vi "Untitled 1.vi"() -> ()   [LabVIEW 2023]
uses:
  Control Timer.ctl
panel:
  out "State":string
  out "RELEASE ALL":bool
  out "MXING":bool
  out "BOILING MILK":bool
  out "ADDING MILK":bool
  out "BOILING":bool
  out "ADDING COFFEE":bool
  out "ADDING WATER":bool
  in  "STOP":bool
  in  "WHITE COFFEE":bool
  in  "CAPUCCINO":bool
  in  "ESPRESSO LONG":bool
  in  "ESPRESSO SHORT":bool
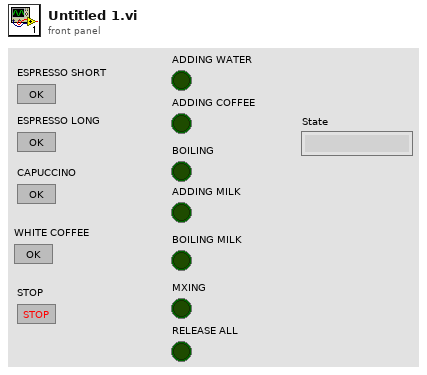
[diagram p1: front panel]
types:
  T1 = typedef "Control Timer.ctl" = enum16{"Timecheck", "Reset"}
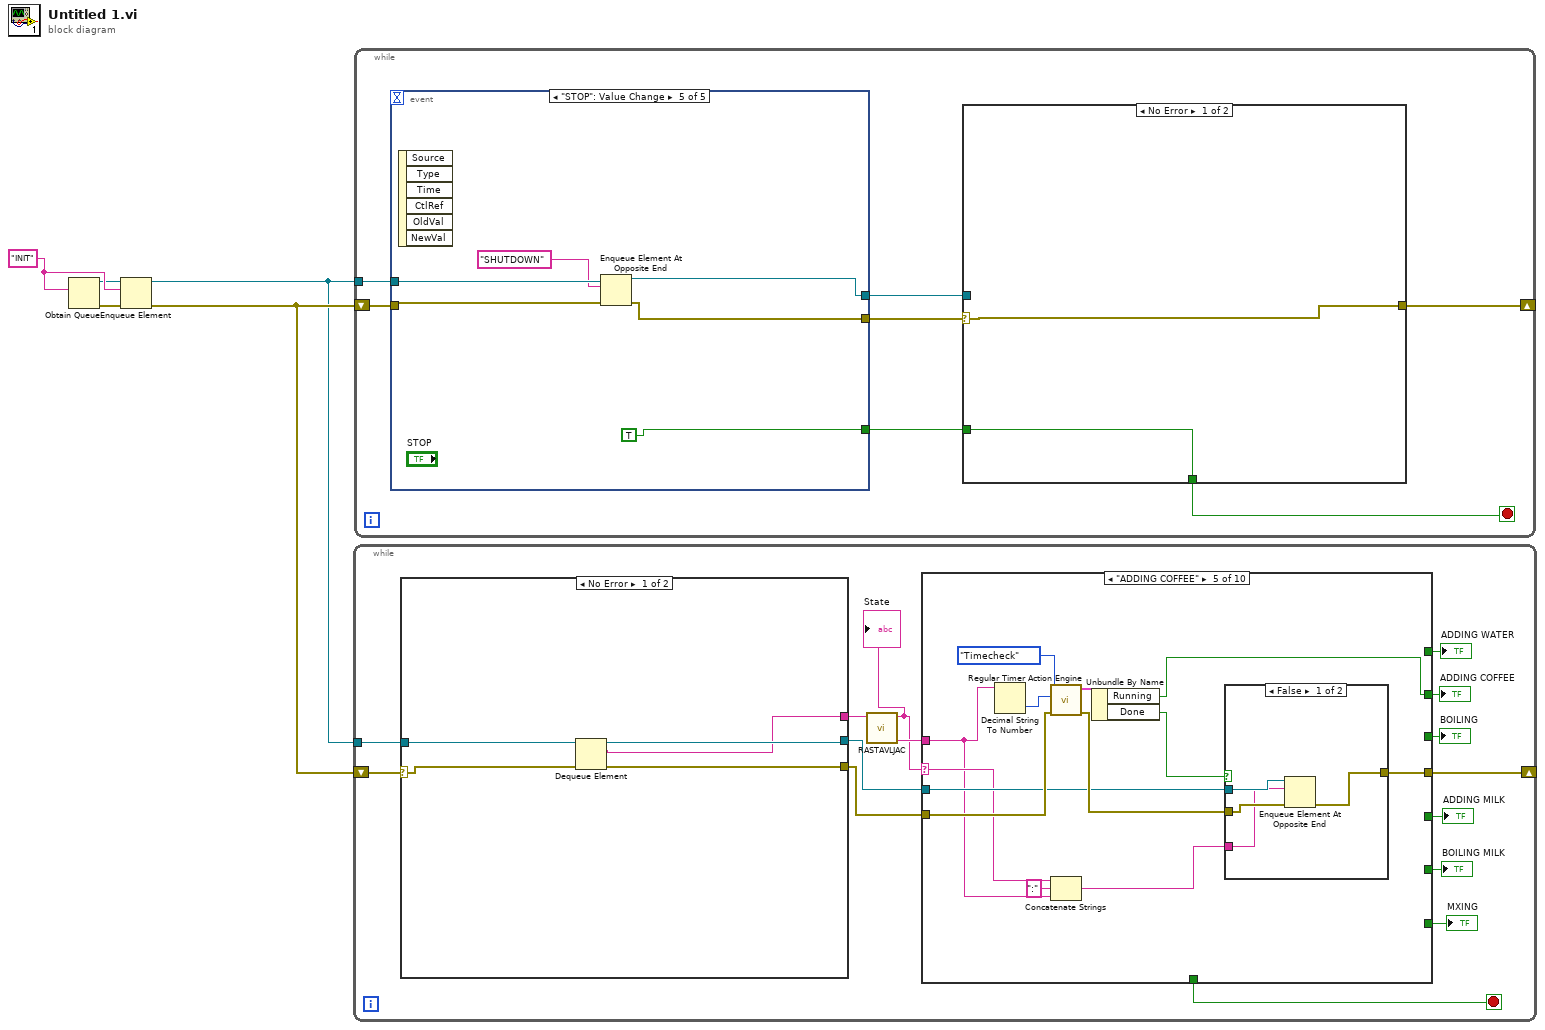
[diagram p0: block diagram]
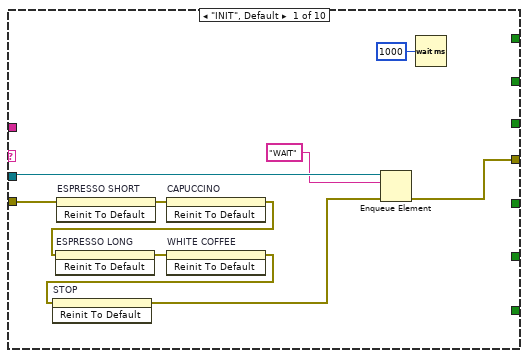
[diagram p2: hidden frame]
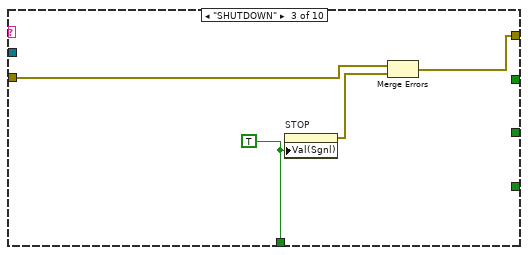
[diagram p4: hidden frame]
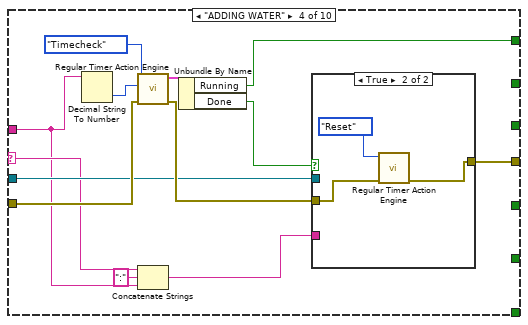
[diagram p5: hidden frame]
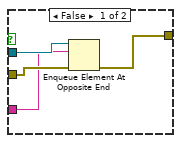
[diagram p6: hidden frame]
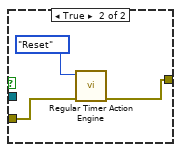
[diagram p7: hidden frame]
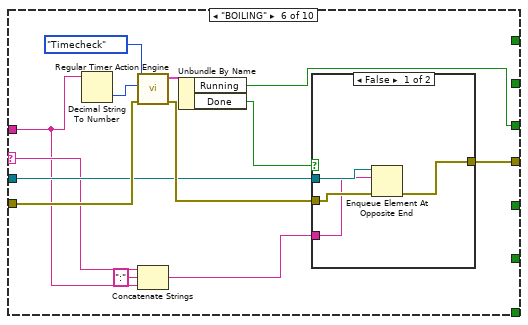
[diagram p8: hidden frame]
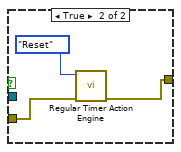
[diagram p9: hidden frame]
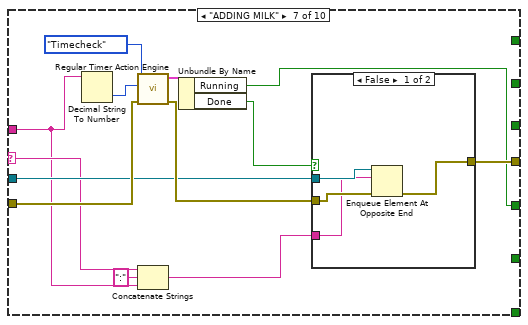
[diagram p10: hidden frame]
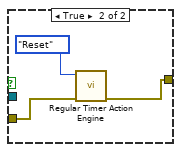
[diagram p11: hidden frame]
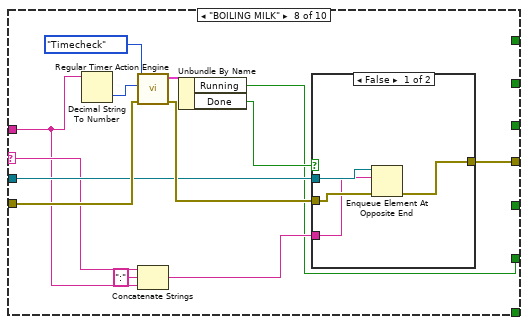
[diagram p12: hidden frame]
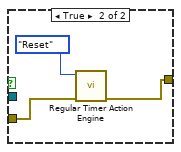
[diagram p13: hidden frame]
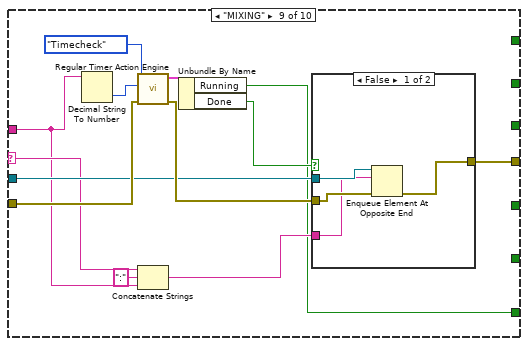
[diagram p14: hidden frame]
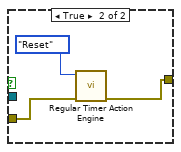
[diagram p15: hidden frame]
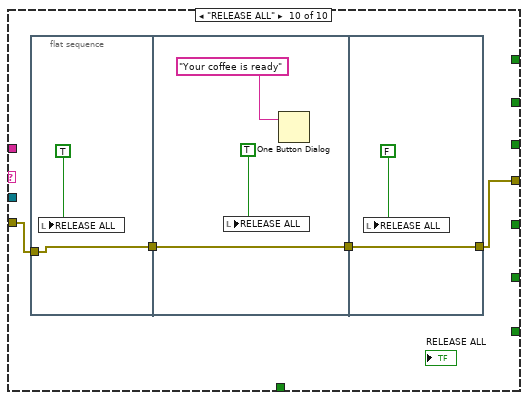
[diagram p16: hidden frame]
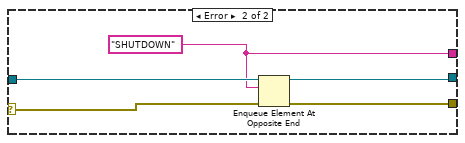
[diagram p17: hidden frame]
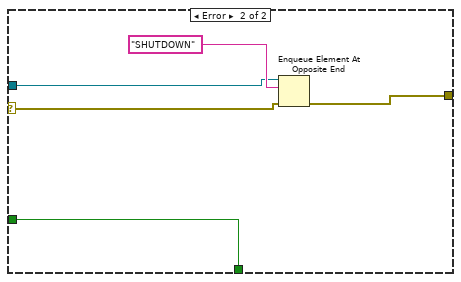
[diagram p18: hidden frame]
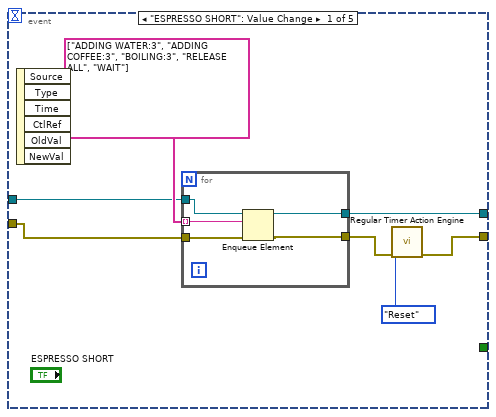
[diagram p19: hidden frame]
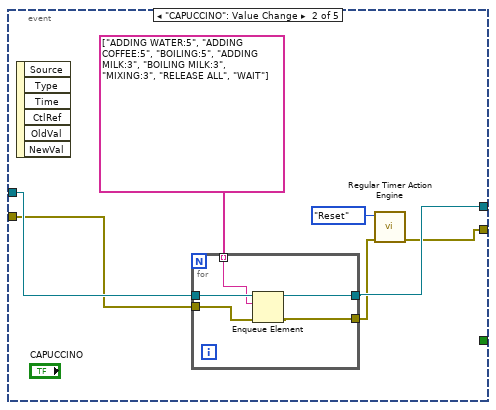
[diagram p20: hidden frame]
diagram:
  w4 = "INIT"
  n1 = Obtain Queue(element data type=w4) -> (queue out=w3:refnum<queue>, error out=w5:errorcluster)  [unwired: 4 in, 1 out]
  n2 = Enqueue Element(queue=w3, element=w4, error in (no error)=w5) -> (queue out=w1:refnum<queue>, error out=w2:errorcluster)  [unwired: 1 in, 1 out]
  n3 = while {
    tunnel: w1 -> [w19]
    shift-right: [w13] -> _
    shift-left: w2 -> [w20]
    stop <- w12 stop-if-true
    n4 = case shown="No Error" w20 {
      selector: w20 -> [w170 w176]
      tunnel: w19 -> [w171 w175]
      tunnel: [w169 w173] -> w15
      tunnel: [w168 w174] -> w14
      tunnel: [w167 w172] -> w18
      frame No Error {
        n5 = Dequeue Element(queue=w171, error in (no error)=w170) -> (queue out=w168:refnum<queue>, element=w167:string, error out=w169:errorcluster)  [unwired: 1 in, 1 out]
      }
      frame Error {
        w172 = "SHUTDOWN"
        n6 = Enqueue Element At Opposite End(queue=w175, element=w172, error in (no error)=w176) -> (queue out=w174:refnum<queue>, error out=w173:errorcluster)  [unwired: 1 in, 1 out]
      }
    }
    n7 = call "RASTAVLJAC.vi"("Input"=w18) -> ("Argument"=w17:string, "State"=w16:string)  [unwired: 9 in]
    "State" <- w16
    n8 = case shown="\"ADDING COFFEE\"" w16 {
      selector: w16 -> [_ _ _ w39 w60 w80 w100 w120 w140 _]
      tunnel: w17 -> [_ _ _ w38 w59 w79 w99 w119 w139 _]
      tunnel: w15 -> [w27 w31 w33 w46 w66 w86 w106 w126 w146 w159]
      tunnel: w14 -> [w30 _ _ w40 w61 w81 w101 w121 w141 _]
      tunnel: [w28 w31 w32 w41 w62 w82 w102 w122 w142 w156] -> w13
      tunnel: [_ _ w35 _ _ _ _ _ _ _] -> w12
      tunnel: [_ _ _ w44 _ _ _ _ _ _] -> w11
      tunnel: [_ _ _ _ w56 _ _ _ _ _] -> w10
      tunnel: [_ _ _ _ _ w76 _ _ _ _] -> w9
      tunnel: [_ _ _ _ _ _ w96 _ _ _] -> w8
      tunnel: [_ _ _ _ _ _ _ w116 _ _] -> w7
      tunnel: [_ _ _ _ _ _ _ _ w136 _] -> w6
      frame "INIT", Default {
        n9 = invoke on="ESPRESSO SHORT" class="Bool" method="Reinit To Default"(error in=w27) -> (error out=w26:errorcluster)  [unwired: 2 in, 2 out]
        n10 = invoke on="CAPUCCINO" class="Bool" method="Reinit To Default"(error in=w26) -> (error out=w25:errorcluster)  [unwired: 2 in, 2 out]
        n11 = invoke on="ESPRESSO LONG" class="Bool" method="Reinit To Default"(error in=w25) -> (error out=w24:errorcluster)  [unwired: 2 in, 2 out]
        n12 = invoke on="WHITE COFFEE" class="Bool" method="Reinit To Default"(error in=w24) -> (error out=w23:errorcluster)  [unwired: 2 in, 2 out]
        n13 = invoke on="STOP" class="Bool" method="Reinit To Default"(error in=w23) -> (error out=w22:errorcluster)  [unwired: 2 in, 2 out]
        n14 = Enqueue Element(queue=w30, element="WAIT", error in (no error)=w22) -> (error out=w28:errorcluster)  [unwired: 1 in, 2 out]
        n15 = Wait (ms)(milliseconds to wait=u32 1000) -> ()  [unwired: 1 out]
      }
      frame "WAIT" {
      }
      frame "SHUTDOWN" {
        w35 = TRUE
        n16 = property on="STOP" class="Bool"("Val(Sgnl)"=w35) -> (error out=w34:errorcluster)  [unwired: 2 in, 1 out]
        n17 = Merge Errors(w33, w34) -> (w32:errorcluster)
      }
      frame "ADDING WATER" {
        n18 = Decimal String To Number(string=w38) -> (number=w48:i32)  [unwired: 2 in, 1 out]
        n19 = call "Regular Timer Action Engine.vi"("Enum"=Control_Timer."Timecheck", "Time Target"=w48, "error in"=w46) -> ("Status"=w45:cluster{"Running":bool, "Done":bool}, "error out"=w42:errorcluster)  [unwired: 6 in]
        n20 = Concatenate Strings(w39, ":" ("string"), w38) -> (w36:string)
        n21 = Unbundle By Name(w45) -> ("Running"=w44:bool, "Done"=w43:bool)
        n22 = case shown="True" w43 {
          tunnel: w42 -> [w51 w55]
          tunnel: [w50 w53] -> w41
          tunnel: w40 -> [w52 _]
          tunnel: w36 -> [w49 _]
          frame False {
            n23 = Enqueue Element At Opposite End(queue=w52, element=w49, error in (no error)=w51) -> (error out=w50:errorcluster)  [unwired: 1 in, 2 out]
          }
          frame True {
            n24 = call "Regular Timer Action Engine.vi"("Enum"=Control_Timer."Reset", "error in"=w55) -> ("error out"=w53:errorcluster)  [unwired: 7 in, 1 out]
          }
        }
      }
      frame "ADDING COFFEE" {
        n25 = Decimal String To Number(string=w59) -> (number=w68:i32)  [unwired: 2 in, 1 out]
        n26 = call "Regular Timer Action Engine.vi"("Enum"=Control_Timer."Timecheck", "Time Target"=w68, "error in"=w66) -> ("Status"=w65:cluster{"Running":bool, "Done":bool}, "error out"=w63:errorcluster)  [unwired: 6 in]
        n27 = Concatenate Strings(w60, ":" ("string"), w59) -> (w57:string)
        n28 = Unbundle By Name(w65) -> ("Running"=w56:bool, "Done"=w64:bool)
        n29 = case shown="False" w64 {
          tunnel: w63 -> [w71 w75]
          tunnel: [w70 w73] -> w62
          tunnel: w61 -> [w72 _]
          tunnel: w57 -> [w69 _]
          frame False {
            n30 = Enqueue Element At Opposite End(queue=w72, element=w69, error in (no error)=w71) -> (error out=w70:errorcluster)  [unwired: 1 in, 2 out]
          }
          frame True {
            n31 = call "Regular Timer Action Engine.vi"("Enum"=Control_Timer."Reset", "error in"=w75) -> ("error out"=w73:errorcluster)  [unwired: 7 in, 1 out]
          }
        }
      }
      frame "BOILING" {
        n32 = Decimal String To Number(string=w79) -> (number=w88:i32)  [unwired: 2 in, 1 out]
        n33 = call "Regular Timer Action Engine.vi"("Enum"=Control_Timer."Timecheck", "Time Target"=w88, "error in"=w86) -> ("Status"=w85:cluster{"Running":bool, "Done":bool}, "error out"=w83:errorcluster)  [unwired: 6 in]
        n34 = Concatenate Strings(w80, ":" ("string"), w79) -> (w77:string)
        n35 = Unbundle By Name(w85) -> ("Running"=w76:bool, "Done"=w84:bool)
        n36 = case shown="False" w84 {
          tunnel: w83 -> [w91 w95]
          tunnel: [w90 w93] -> w82
          tunnel: w81 -> [w92 _]
          tunnel: w77 -> [w89 _]
          frame False {
            n37 = Enqueue Element At Opposite End(queue=w92, element=w89, error in (no error)=w91) -> (error out=w90:errorcluster)  [unwired: 1 in, 2 out]
          }
          frame True {
            n38 = call "Regular Timer Action Engine.vi"("Enum"=Control_Timer."Reset", "error in"=w95) -> ("error out"=w93:errorcluster)  [unwired: 7 in, 1 out]
          }
        }
      }
      frame "ADDING MILK" {
        n39 = Decimal String To Number(string=w99) -> (number=w108:i32)  [unwired: 2 in, 1 out]
        n40 = call "Regular Timer Action Engine.vi"("Enum"=Control_Timer."Timecheck", "Time Target"=w108, "error in"=w106) -> ("Status"=w105:cluster{"Running":bool, "Done":bool}, "error out"=w103:errorcluster)  [unwired: 6 in]
        n41 = Concatenate Strings(w100, ":" ("string"), w99) -> (w97:string)
        n42 = Unbundle By Name(w105) -> ("Running"=w96:bool, "Done"=w104:bool)
        n43 = case shown="False" w104 {
          tunnel: w103 -> [w111 w115]
          tunnel: [w110 w113] -> w102
          tunnel: w101 -> [w112 _]
          tunnel: w97 -> [w109 _]
          frame False {
            n44 = Enqueue Element At Opposite End(queue=w112, element=w109, error in (no error)=w111) -> (error out=w110:errorcluster)  [unwired: 1 in, 2 out]
          }
          frame True {
            n45 = call "Regular Timer Action Engine.vi"("Enum"=Control_Timer."Reset", "error in"=w115) -> ("error out"=w113:errorcluster)  [unwired: 7 in, 1 out]
          }
        }
      }
      frame "BOILING MILK" {
        n46 = Decimal String To Number(string=w119) -> (number=w128:i32)  [unwired: 2 in, 1 out]
        n47 = call "Regular Timer Action Engine.vi"("Enum"=Control_Timer."Timecheck", "Time Target"=w128, "error in"=w126) -> ("Status"=w125:cluster{"Running":bool, "Done":bool}, "error out"=w123:errorcluster)  [unwired: 6 in]
        n48 = Concatenate Strings(w120, ":" ("string"), w119) -> (w117:string)
        n49 = Unbundle By Name(w125) -> ("Running"=w116:bool, "Done"=w124:bool)
        n50 = case shown="False" w124 {
          tunnel: w123 -> [w131 w135]
          tunnel: [w130 w133] -> w122
          tunnel: w121 -> [w132 _]
          tunnel: w117 -> [w129 _]
          frame False {
            n51 = Enqueue Element At Opposite End(queue=w132, element=w129, error in (no error)=w131) -> (error out=w130:errorcluster)  [unwired: 1 in, 2 out]
          }
          frame True {
            n52 = call "Regular Timer Action Engine.vi"("Enum"=Control_Timer."Reset", "error in"=w135) -> ("error out"=w133:errorcluster)  [unwired: 7 in, 1 out]
          }
        }
      }
      frame "MIXING" {
        n53 = Decimal String To Number(string=w139) -> (number=w148:i32)  [unwired: 2 in, 1 out]
        n54 = call "Regular Timer Action Engine.vi"("Enum"=Control_Timer."Timecheck", "Time Target"=w148, "error in"=w146) -> ("Status"=w145:cluster{"Running":bool, "Done":bool}, "error out"=w143:errorcluster)  [unwired: 6 in]
        n55 = Concatenate Strings(w140, ":" ("string"), w139) -> (w137:string)
        n56 = Unbundle By Name(w145) -> ("Running"=w136:bool, "Done"=w144:bool)
        n57 = case shown="False" w144 {
          tunnel: w143 -> [w151 w155]
          tunnel: [w150 w153] -> w142
          tunnel: w141 -> [w152 _]
          tunnel: w137 -> [w149 _]
          frame False {
            n58 = Enqueue Element At Opposite End(queue=w152, element=w149, error in (no error)=w151) -> (error out=w150:errorcluster)  [unwired: 1 in, 2 out]
          }
          frame True {
            n59 = call "Regular Timer Action Engine.vi"("Enum"=Control_Timer."Reset", "error in"=w155) -> ("error out"=w153:errorcluster)  [unwired: 7 in, 1 out]
          }
        }
      }
      frame "RELEASE ALL" {
        n60 = flat-sequence {
          tunnel: w159 -> [w160]
          tunnel: [w160] -> w157
          tunnel: [w162] -> w158
          tunnel: w157 -> [w162]
          tunnel: [w165] -> w156
          tunnel: w158 -> [w165]
          frame #0 {
            n61 = local write "RELEASE ALL"(TRUE ("RELEASE ALL")) -> ()
          }
          frame #1 {
            n62 = local write "RELEASE ALL"(TRUE ("RELEASE ALL")) -> ()
            n63 = One Button Dialog(message="Your coffee is ready") -> ()  [unwired: 1 in, 1 out]
          }
          frame #2 {
            n64 = local write "RELEASE ALL"(FALSE ("RELEASE ALL")) -> ()
          }
        }
      }
    }
    "ADDING WATER" <- w11
    "ADDING COFFEE" <- w10
    "BOILING" <- w9
    "ADDING MILK" <- w8
    "BOILING MILK" <- w7
    "MXING" <- w6
  }
  n65 = while {
    tunnel: w1 -> [w183]
    shift-right: [w178] -> _
    shift-left: w2 -> [w182]
    stop <- w177 stop-if-true
    n66 = event shown="[4] \"STOP\": Value Change" {
      selector: _ -> [_ _ _ _ _]
      dyn-events: _ -> [_ _ _ _ _]
      timeout: _ -> [_ _ _ _ _]
      tunnel: w183 -> [w196 w209 w220 w232 w241]
      tunnel: w182 -> [w195 w208 w219 w231 w240]
      tunnel: [w194 w206 w221 w233 w242] -> w179
      tunnel: [w192 w204 w216 w228 w243] -> w181
      tunnel: [_ _ _ _ TRUE] -> w180
      event "ESPRESSO SHORT": Value Change {
        n67 = event-data() -> ()  [unwired: 1 in, 6 out]
        n68 = for {
          tunnel: string[] ["ADDING WATER:3", "ADDING COFFEE:3", "BOILING:3", "RELEASE ALL", "WAIT"] -> [w202] mode=indexing
          tunnel: [w201] -> w194
          tunnel: [w200] -> w193
          tunnel: w196 -> [w199]
          tunnel: w195 -> [w198]
          n69 = Enqueue Element(queue=w199, element=w202, error in (no error)=w198) -> (queue out=w201:refnum<queue>, error out=w200:errorcluster)  [unwired: 1 in, 1 out]
        }
        n70 = call "Regular Timer Action Engine.vi"("Enum"=Control_Timer."Reset", "error in"=w193) -> ("error out"=w192:errorcluster)  [unwired: 7 in, 1 out]
      }
      event "CAPUCCINO": Value Change {
        n71 = event-data() -> ()  [unwired: 1 in, 6 out]
        n72 = for {
          tunnel: [w214] -> w206
          tunnel: [w213] -> w205
          tunnel: w209 -> [w212]
          tunnel: w208 -> [w211]
          tunnel: string[] ["ADDING WATER:5", "ADDING COFFEE:5", "BOILING:5", "ADDING MILK:3", "BOILING MILK:3", "MIXING:3", "RELEASE ALL", "WAIT"] -> [w210] mode=indexing
          n73 = Enqueue Element(queue=w212, element=w210, error in (no error)=w211) -> (queue out=w214:refnum<queue>, error out=w213:errorcluster)  [unwired: 1 in, 1 out]
        }
        n74 = call "Regular Timer Action Engine.vi"("Enum"=Control_Timer."Reset", "error in"=w205) -> ("error out"=w204:errorcluster)  [unwired: 7 in, 1 out]
      }
      event "ESPRESSO LONG": Value Change {
        n75 = event-data() -> ()  [unwired: 1 in, 6 out]
        n76 = for {
          tunnel: [w226] -> w221
          tunnel: [w225] -> w217
          tunnel: w220 -> [w224]
          tunnel: w219 -> [w223]
          tunnel: string[] ["ADDING WATER:5", "ADDING COFFEE:5", "BOILING:5", "RELEASE ALL", "WAIT"] -> [w222] mode=indexing
          n77 = Enqueue Element(queue=w224, element=w222, error in (no error)=w223) -> (queue out=w226:refnum<queue>, error out=w225:errorcluster)  [unwired: 1 in, 1 out]
        }
        n78 = call "Regular Timer Action Engine.vi"("Enum"=Control_Timer."Reset", "error in"=w217) -> ("error out"=w216:errorcluster)  [unwired: 7 in, 1 out]
      }
      event "WHITE COFFEE": Value Change {
        n79 = event-data() -> ()  [unwired: 1 in, 6 out]
        n80 = for {
          tunnel: [w238] -> w233
          tunnel: [w237] -> w229
          tunnel: w232 -> [w236]
          tunnel: w231 -> [w235]
          tunnel: string[] ["ADDING MILK:5", "ADDING COFFEE:2", "BOILING MILK:3", "RELEASE ALL", "WAIT"] -> [w234] mode=indexing
          n81 = Enqueue Element(queue=w236, element=w234, error in (no error)=w235) -> (queue out=w238:refnum<queue>, error out=w237:errorcluster)  [unwired: 1 in, 1 out]
        }
        n82 = call "Regular Timer Action Engine.vi"("Enum"=Control_Timer."Reset", "error in"=w229) -> ("error out"=w228:errorcluster)  [unwired: 7 in, 1 out]
      }
      event "STOP": Value Change {
        n83 = event-data() -> ()  [unwired: 1 in, 6 out]
        n84 = Enqueue Element At Opposite End(queue=w241, element="SHUTDOWN", error in (no error)=w240) -> (queue out=w242:refnum<queue>, error out=w243:errorcluster)  [unwired: 1 in, 1 out]
      }
    }
    n85 = case shown="No Error" w181 {
      selector: w181 -> [w185 w189]
      tunnel: w180 -> [w184 w186]
      tunnel: w179 -> [_ w188]
      tunnel: [w185 w187] -> w178
      tunnel: [w184 w186] -> w177
      frame No Error {
      }
      frame Error {
        n86 = Enqueue Element At Opposite End(queue=w188, element="SHUTDOWN", error in (no error)=w189) -> (error out=w187:errorcluster)  [unwired: 1 in, 2 out]
      }
    }
  }
